vi "Actor Core.vi"(8 "error in":errorcluster, 11 "Nested in":refnum<class "Generador de Funciones.lvclass">) -> (0 "error out":errorcluster, 3 "Actor out":refnum<class "Actor.lvclass">)   [LabVIEW 2020, in "Generador de Funciones.lvlib" / "Generador de Funciones.lvclass"]
doc: "(<B>Filename</B>: Actor Framework.lvlib:Actor.lvclass:Actor Core.vi)\n\nReceives messages to the actor, reacts to them, and initiates any error handling that may shut the actor down.\n\nDescendant classes may override this VI to append parallel tasks for the actor to complete while it handles messages. Overrides use the Call Parent Method node."
uses:
  Generador de Funciones.lvclass
  C:/Program Files (x86)/National Instruments/LabVIEW 2020/vi.lib/ActorFramework/Actor/Actor.lvclass
  <vilib>/ActorFramework/Actor/Actor.lvclass
  <vilib>/ActorFramework/Actor/Actor.lvclass/Actor.ctl
  <vilib>/ActorFramework/Message Enqueuer/Message Enqueuer.lvclass/Message Enqueuer.ctl
  Generador de Funciones.lvclass/Generador de Funciones.ctl
  Generador de Funciones Messages/Amplitud Msg/Amplitud Msg.lvclass/Amplitud Msg.ctl
  Generador de Funciones Messages/Frecuencia Msg/Frecuencia Msg.lvclass/Frecuencia Msg.ctl
  <vilib>/ActorFramework/Message Enqueuer/Init from Existing Queue.vi
  <vilib>/ActorFramework/Message Enqueuer/Enqueue.vi
  <vilib>/ActorFramework/Stop Msg/Stop Msg.lvclass
  C:/Program Files (x86)/National Instruments/LabVIEW 2020/vi.lib/ActorFramework/Message/Message.lvclass
  Generador de Funciones Messages/Graph Data Msg/Graph Data Msg.lvclass
  Generador de Funciones Messages/Amplitud Msg/Amplitud Msg.lvclass
  Generador de Funciones Messages/Frecuencia Msg/Frecuencia Msg.lvclass
  <vilib>/ActorFramework/Message Priority Queue/Priority Enqueue.vi
  <vilib>/ActorFramework/Message Enqueuer/Message Enqueuer.lvclass
panel:
  out "Waveform Graph":dbl[](graph)
  in  "Path":path
  in  "Exit":bool
  in  "Tipo de señal":enum16{"Cuadrada", "Triangular", "Senoidal"}(ring)
  in  "Guardar datos":bool
  in  "Stop":bool
  in  "Start":bool
  in  "Frecuencia":dbl
  in  "Amplitud":dbl
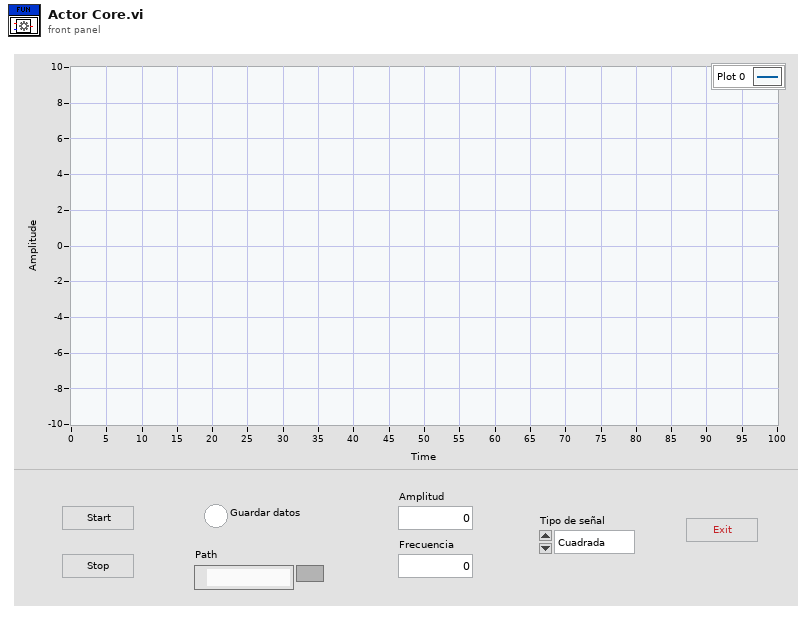
[diagram p1: front panel]
types:
  T1 = cluster{"Stop":refnum<user-event>, "Waveform Chart":refnum<user-event>, "Waveform Graph":refnum<user-event>}
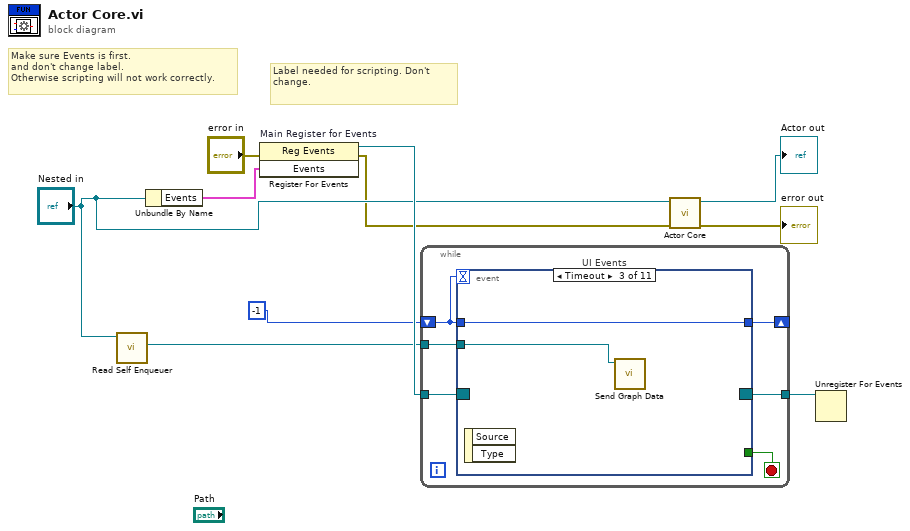
[diagram p0: block diagram]
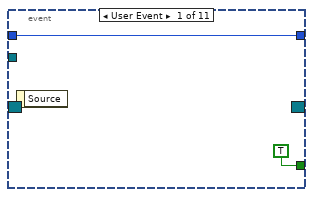
[diagram p2: hidden frame]
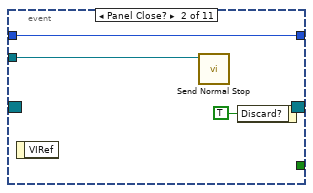
[diagram p3: hidden frame]
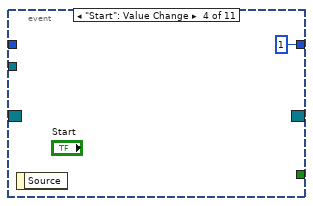
[diagram p4: hidden frame]
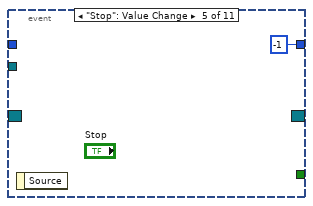
[diagram p5: hidden frame]
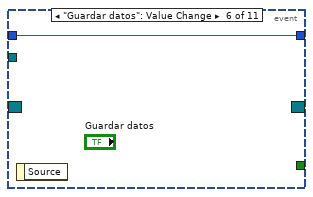
[diagram p6: hidden frame]
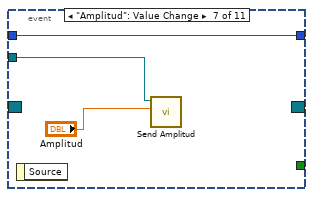
[diagram p7: hidden frame]
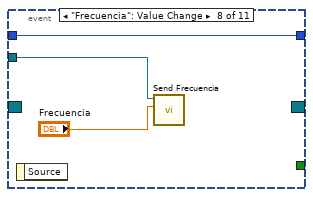
[diagram p8: hidden frame]
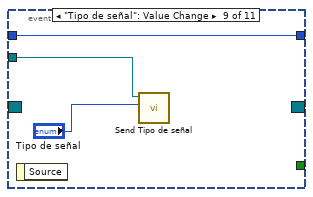
[diagram p9: hidden frame]
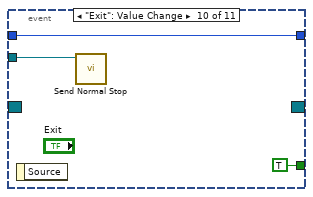
[diagram p10: hidden frame]
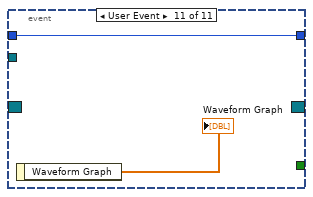
[diagram p11: hidden frame]
diagram:
  # "Label needed for scripting. Don't change."
  # "Make sure Events is first.\nand don't change label.\nOtherwise scripting will not work correctly."
  n1 = call <vilib>:"Read Self Enqueuer.vi"("Actor"="Nested in") -> ("Self Enqueuer"=w4:refnum<class "Message Enqueuer.lvclass">)  [unwired: 10 in]
  n2 = Unbundle By Name("Nested in") -> ("Events"=w7:T1)
  n3 = register-events "Main Register for Events"(error in="error in", w7) -> (reference out=w8:refnum<event-registration>, error out=w2:errorcluster)  [unwired: 1 in]
  n4 = while {
    tunnel: w8 -> [w16]
    tunnel: [w14] -> w6
    tunnel: w4 -> [w13]
    shift-right: [w11] -> _
    shift-left: -1 -> [w12]
    stop <- w15 stop-if-true
    n5 = event "UI Events" shown="[2] Timeout" {
      selector: w16 -> [_ _ _ _ _ _ _ _ _ _ _]
      dyn-events: [_ _ _ _ _ _ _ _ _ _ _] -> w14
      timeout: w12 -> [_ _ _ _ _ _ _ _ _ _ _]
      tunnel: [TRUE _ _ _ _ _ _ _ _ TRUE _] -> w15
      tunnel: w13 -> [_ w20 w22 _ _ _ w28 w31 w34 w38 _]
      tunnel: w12 -> [w17 w19 w23 _ _ w26 w29 w32 w35 w36 w40]
      tunnel: [w17 w19 w23 1 -1 w26 w29 w32 w35 w36 w40] -> w11
      event User Event {
        n6 = event-data() -> ()  [unwired: 1 in, 1 out]
      }
      event Panel Close? {
        n7 = event-data() -> ()  [unwired: 1 in, 1 out]
        n8 = call <vilib>:"Send Normal Stop.vi"("Message Enqueuer"=w20) -> ()  [unwired: 10 in, 1 out]
        n9 = event-data("Discard?"=TRUE) -> ()  [unwired: 1 in, 1 out]
      }
      event Timeout {
        n10 = event-data() -> ()  [unwired: 1 in, 2 out]
        n11 = call "Send Graph Data.vi"("Message Enqueuer"=w22) -> ()  [unwired: 9 in, 2 out]
      }
      event "Start": Value Change {
        n12 = event-data() -> ()  [unwired: 1 in, 1 out]
      }
      event "Stop": Value Change {
        n13 = event-data() -> ()  [unwired: 1 in, 1 out]
      }
      event "Guardar datos": Value Change {
        n14 = event-data() -> ()  [unwired: 1 in, 1 out]
      }
      event "Amplitud": Value Change {
        n15 = event-data() -> ()  [unwired: 1 in, 1 out]
        n16 = call "Send Amplitud.vi"("Numeric"="Amplitud", "Message Enqueuer"=w28) -> ()  [unwired: 8 in, 2 out]
      }
      event "Frecuencia": Value Change {
        n17 = event-data() -> ()  [unwired: 1 in, 1 out]
        n18 = call "Send Frecuencia.vi"("Numeric"="Frecuencia", "Message Enqueuer"=w31) -> ()  [unwired: 8 in, 2 out]
      }
      event "Tipo de señal": Value Change {
        n19 = event-data() -> ()  [unwired: 1 in, 1 out]
        n20 = call "Send Tipo de señal.vi"("Tipo de señal"="Tipo de señal", "Message Enqueuer"=w34) -> ()  [unwired: 8 in, 2 out]
      }
      event "Exit": Value Change {
        n21 = event-data() -> ()  [unwired: 1 in, 1 out]
        n22 = call <vilib>:"Send Normal Stop.vi"("Message Enqueuer"=w38) -> ()  [unwired: 10 in, 1 out]
      }
      event User Event {
        n23 = event-data() -> ("Waveform Graph"=→"Waveform Graph":dbl[])  [unwired: 1 in]
      }
    }
  }
  n24 = call-parent "Actor Core.vi"("error in"=w2, "Actor in"="Nested in") -> ("error out"=→"error out":errorcluster, "Actor out"=→"Actor out":refnum<class "Actor.lvclass">)  [unwired: 8 in]
  n25 = Unregister For Events(event registration refnum=w6) -> ()  [unwired: 1 in, 1 out]
